vi "Get Resource Identifier.vi"(8 "Error In":errorcluster, 11 "object in":refnum<class "Continuous Waveform Acq CFG.lvclass">) -> (0 "Error Out":errorcluster, 2 "instrument handle":refnum<k15>, 3 "object out":refnum<class "Continuous Waveform Acq CFG.lvclass">)   [LabVIEW 2023, in "PXIe-5172 Simulated.lvlib" / "Continuous Waveform Acq CFG.lvclass"]
uses:
  Continuous Waveform Acq CFG.lvclass
  Continuous Waveform Acq CFG.lvclass/Continuous Waveform Acq CFG.ctl
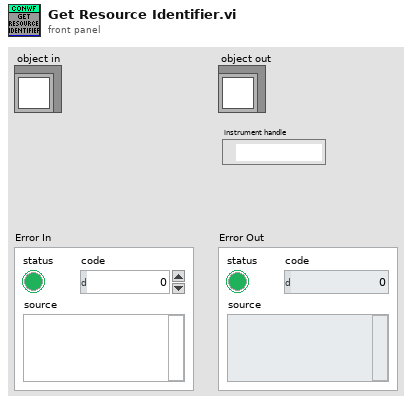
[diagram p1: front panel]
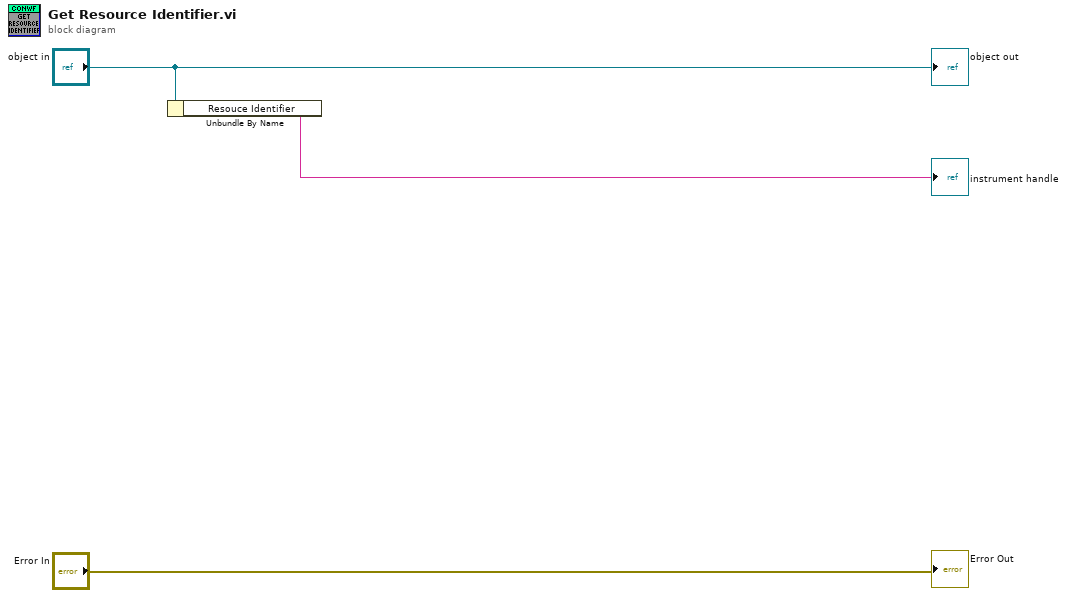
[diagram p0: block diagram]
diagram:
  n1 = Unbundle By Name("object in") -> ("Resouce Identifier"=→"instrument handle":string)
  "Error Out" <- "Error In"
  "object out" <- "object in"
